vi "PagesUI.vi"() -> ()   [LabVIEW 2015, in "Pages.lvclass"]
uses:
  Pages.lvclass
  <vilib>/NI/Configuration Framework/Node/NodeRef.ctl
  <vilib>/NI/Configuration Framework/Node/NISE_CEF_Node.lvclass
  <vilib>/NI/AMC/Message Queue.ctl
  <vilib>/NI/AMC/Message.ctl
  <vilib>/NI/Tools/Keyed Array/KeyedArray.ctl
  <vilib>/NI/Configuration Framework/Node/UserEventRef.ctl
  <vilib>/NI/Configuration Framework/Controls/EventCluster.ctl
  <vilib>/Utility/sysdir.llb/System Directory Type.ctl
  subVI/Config Global.vi
  <vilib>/NI/AMC/AMC.lvlib
  Configuration Tool.lvlib
  <vilib>/NI/Tools/Keyed Array/Tools_KeyedArray.lvlib
  <vilib>/NI/Configuration Framework/NISE_CEF_TreeControl.lvlib
panel:
  in  "WebBrowser":refnum<k7>(container)
  in  "user event":T1
  in  "main queue":T2
  in  "node ref":T3
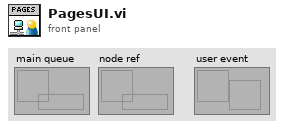
[diagram p1: front panel]
types:
  T1 = typedef "NISE_CEF_Node.lvclass/UserEventRef.ctl" = refnum<user-event>
  T2 = typedef "AMC.lvlib/Message Queue.ctl" = refnum<queue>
  T3 = typedef "NISE_CEF_Node.lvclass/NodeRef.ctl" = refnum<data-value>
  T4 = typedef "System Directory Type.ctl" = i32
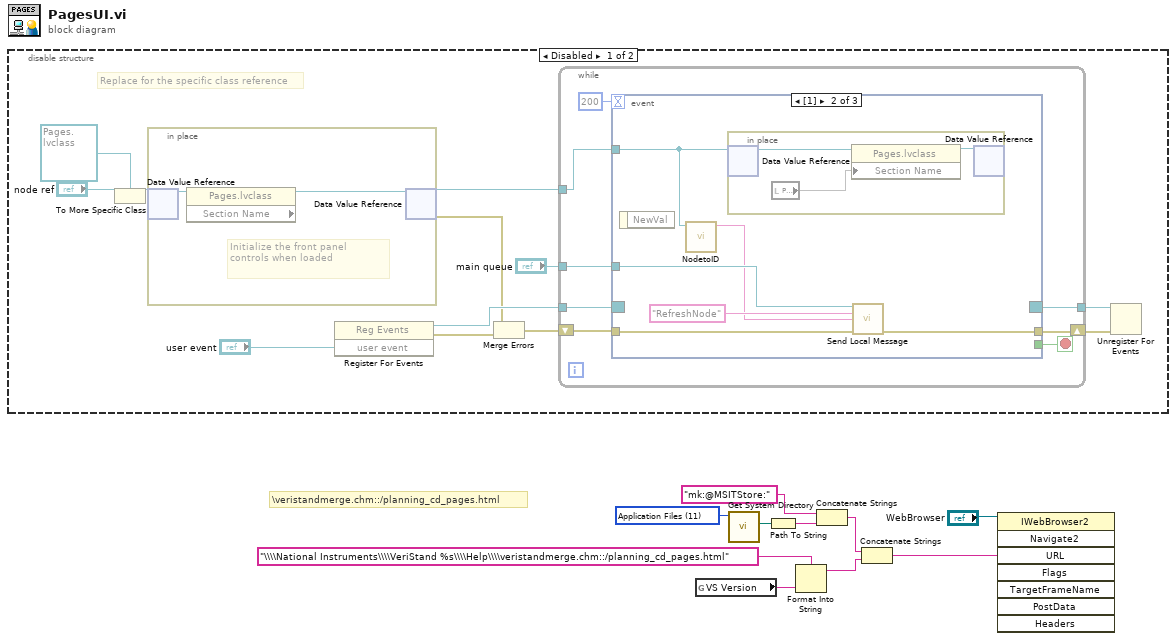
[diagram p0: block diagram]
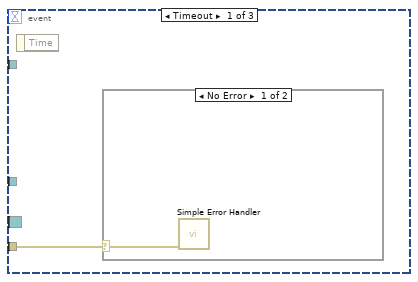
[diagram p2: hidden frame]
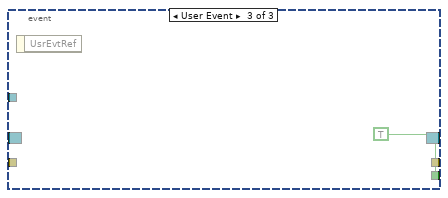
[diagram p4: hidden frame]
diagram:
  w10 = T4 11 items=["User Home"=0, "User Desktop"=1, "User Documents"=2, "User Application Data"=3, "User Preferences"=4, "User Temporary"=5, "Public Documents"=6, "Public Application Data"=7, "Public Preferences"=8, "Public Cache"=13, "System Core Libraries"=9, "System Installed Libraries"=10, "Application Files"=11, "Boot Volume Root"=12] ("system directory type")
  # "\\veristandmerge.chm::/planning_cd_pages.html"
  n1 = disable-structure shown="Disabled" {
    frame Disabled {
      # "Replace for the specific class reference"
      n2 = To More Specific Class(target class=refnum<data-value> refnum ("data value reference"), reference="node ref") -> (specific class reference=w15:refnum<data-value>)  [unwired: 1 in, 1 out]
      n3 = in-place {
        # "Initialize the front panel controls when loaded"
        n4 = in-place-dvr #1(w15) -> (w45:refnum<class "Pages.lvclass">)  [unwired: 1 out]
        n5 = property class="Pages.lvclass"(reference=w45) -> (reference out=w44:refnum<class "Pages.lvclass">, "Section Name"=w43:string)  [unwired: 1 in, 1 out]
        n6 = in-place-dvr #1(w44) -> (w22:refnum<data-value>, w12:errorcluster)
      }
      n7 = register-events("user event") -> (reference out=w19:refnum<event-registration>, error out=w13:errorcluster)  [unwired: 2 in]
      n8 = Merge Errors(w12, w13) -> (w11:errorcluster)
      n9 = while {
        tunnel: w22 -> [w30]
        tunnel: "main queue" -> [w29]
        tunnel: w19 -> [w27]
        tunnel: [w26] -> w18
        shift-right: [w24] -> w17
        shift-left: w11 -> [w23]
        stop <- w25 stop-if-true
        n10 = event shown="[1]" {
          selector: w27 -> [_ _ _]
          dyn-events: [_ _ _] -> w26
          timeout: 200 -> [_ _ _]
          tunnel: w30 -> [_ w36 _]
          tunnel: w29 -> [_ w37 _]
          tunnel: [_ _ TRUE] -> w25
          tunnel: [_ w34 _] -> w24
          tunnel: w23 -> [w31 w33 _]
          event Timeout {
            n11 = event-data() -> ()  [unwired: 1 in, 1 out]
            n12 = case shown="No Error" w31 {
              selector: w31 -> [w32 _]
              frame No Error {
                n13 = call <vilib>:"Simple Error Handler.vi"("error in (no error)"=w32) -> ()  [unwired: 4 in, 5 out]
              }
              frame Error {
              }
            }
          }
          event #1 (no event record) {
            n14 = event-data() -> ()  [unwired: 1 in, 1 out]
            n15 = call <vilib>:"NodetoID.vi"("node ref"=w36) -> ("ID"=w35:string)  [unwired: 9 in, 1 out]
            n16 = in-place {
              n17 = in-place-dvr #2(w36) -> (w41:refnum<class "Pages.lvclass">)  [unwired: 1 out]
              n18 = local read item#-1() -> (w39)
              n19 = property class="Pages.lvclass"(reference=w41, "Section Name"=w39) -> (reference out=w40:refnum<class "Pages.lvclass">)  [unwired: 1 in, 1 out]
              n20 = in-place-dvr #2(w40) -> ()  [unwired: 2 out]
            }
            n21 = call <vilib>:"Send Local Message.vi"("message queue in"=w37, "message name"="RefreshNode" ("Message Name"), "message value"=w35, "error in"=w33) -> ("error out"=w34:errorcluster)  [unwired: 9 in, 2 out]
          }
          event User Event {
            n22 = event-data() -> ()  [unwired: 1 in, 1 out]
          }
        }
      }
      n23 = Unregister For Events(event registration refnum=w18, error in=w17) -> ()  [unwired: 1 out]
    }
    frame Enabled {
    }
  }
  n24 = global read "Config Global.vi" "VS Version"() -> (w3:string)
  n25 = call <vilib>:"Get System Directory.vi"("system directory type"=w10) -> ("system directory"=w9:path)  [unwired: 10 in]
  n26 = Path To String(path=w9) -> (string=w8:string)
  n27 = Format Into String(format string="\\\\National Instruments\\\\VeriStand %s\\\\Help\\\\veristandmerge.chm::/planning_cd_pages.html", w3) -> (resulting string=w5:string)  [unwired: 2 in, 1 out]
  n28 = Concatenate Strings("mk:@MSITStore:" ("concatenated string"), w8) -> (w6:string)
  n29 = Concatenate Strings(w6, w5) -> (w2:string)
  n30 = invoke class="IWebBrowser2" method="Navigate2"(reference="WebBrowser", "URL"=w2) -> ()  [unwired: 6 in, 8 out]
